vi "调频信号与解调.vi"() -> ()   [LabVIEW 2018]
panel:
  in  "噪声幅度":dbl(slide) min=0.0 max=5.0 scale=0.0..5.0
  out "调制后时域波形":dynamicdata(graph)
  out "发送数据":i32[](array[numeric])
  out "解码正确":bool
  in  "停止":bool
  out "接收数据":dbl[](array[numeric])
  out "滤波后波形":dynamicdata(graph)
  out "相干后波形":dynamicdata(graph)
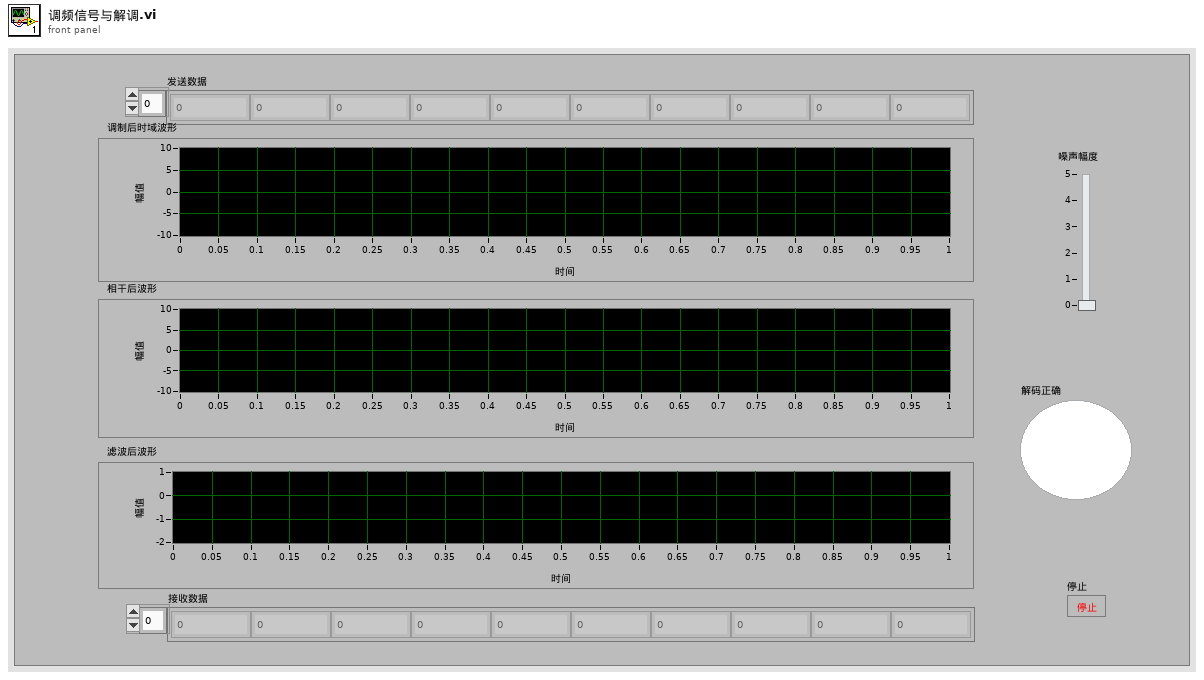
[diagram p1: front panel]
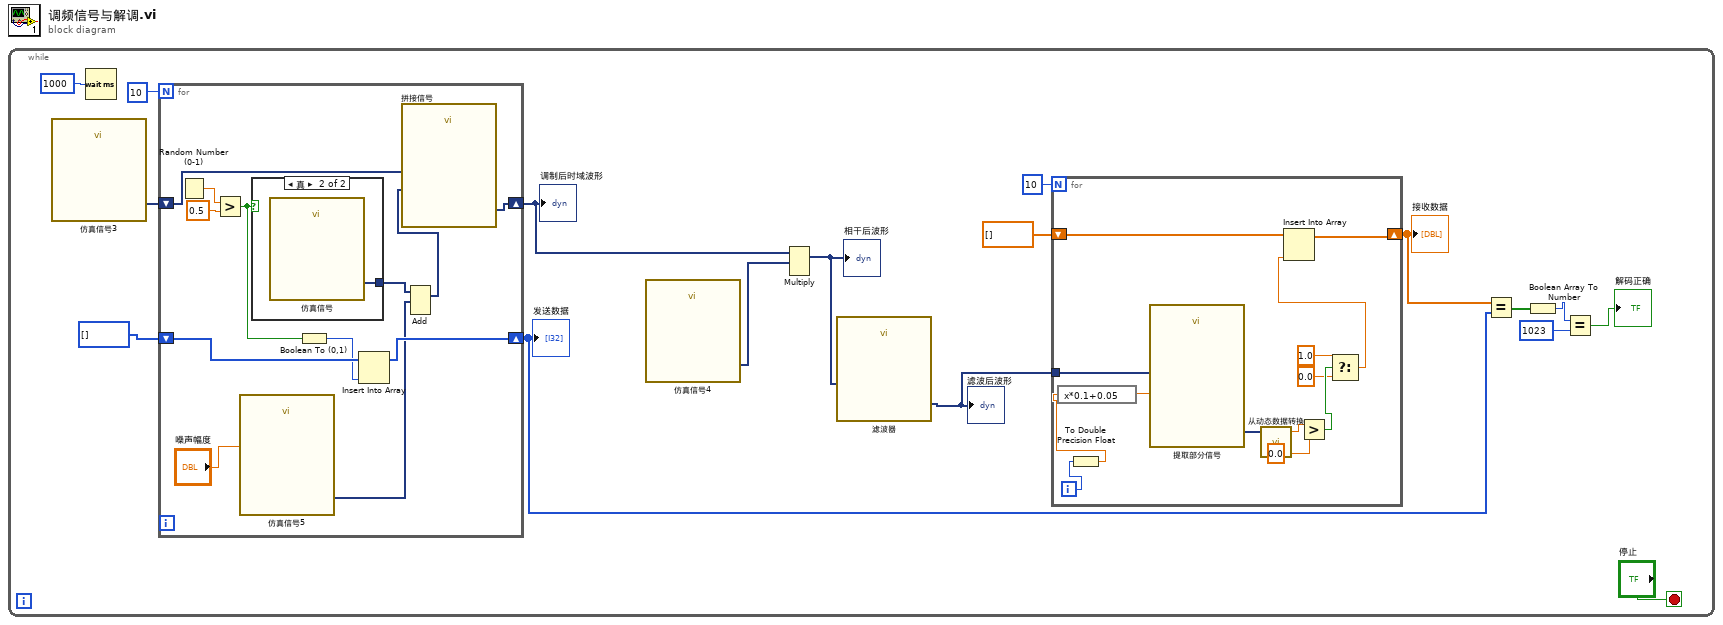
[diagram p0: block diagram]
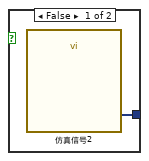
[diagram p2: hidden frame]
diagram:
  n1 = while {
    stop <- "停止" stop-if-true
    n2 = call "仿真信号3"() -> ("正弦"=w16:dynamicdata)  [unwired: 14 in, 1 out]
    n3 = Wait (ms)(milliseconds to wait=u32 1000 ("等待时间（毫秒）")) -> ()  [unwired: 1 out]
    n4 = for {
      N: 10 -> [_]
      shift-right: [w40] -> w11
      shift-left: w16 -> [w39]
      shift-right: [w35] -> w5
      shift-left: i32[] [] -> [w37]
      n5 = Random Number (0-1)() -> (number: 0 to 1=w41:dbl)
      n6 = Greater?(x=w41, y=0.5) -> (0:w38:bool)
      n7 = call "仿真信号5"("噪声幅值"="噪声幅度") -> ("正弦与均匀噪声"=w33:dynamicdata)  [unwired: 13 in, 1 out]
      n8 = case shown="真" w38 {
        tunnel: [w43 w44] -> w32
        frame False {
          n9 = call "仿真信号2"() -> ("正弦"=w43:dynamicdata)  [unwired: 14 in, 1 out]
        }
        frame True {
          n10 = call "仿真信号"() -> ("正弦"=w44:dynamicdata)  [unwired: 14 in, 1 out]
        }
      }
      n11 = Boolean To (0,1)(Boolean=w38) -> (0, 1=w36:i16)
      n12 = Insert Into Array(array=w37, new element=w36) -> (w35:i32[])  [unwired: 1 in]
      n13 = Add(1:w33, 2:w32) -> (0:w31:dynamicdata)  [unwired: 1 in, 1 out]
      n14 = call "拼接信号"("Input Signal B"=w31, "Input Signal A"=w39) -> ("Appended Signals"=w40:dynamicdata)  [unwired: 8 in, 1 out]
    }
    "调制后时域波形" <- w11
    "发送数据" <- w5
    n15 = call "仿真信号4"() -> ("正弦"=w12:dynamicdata)  [unwired: 14 in, 1 out]
    n16 = Multiply(1:w12, 2:w11) -> (0:w10:dynamicdata)  [unwired: 1 in, 1 out]
    "相干后波形" <- w10
    n17 = call "滤波器"("Signal"=w10) -> ("Filtered Signal"=w8:dynamicdata)  [unwired: 9 in, 1 out]
    "滤波后波形" <- w8
    n18 = for {
      N: 10 -> [_]
      tunnel: w8 -> [w30]
      shift-right: [w24] -> w6
      shift-left: dbl[] [] -> [w25]
      i -> [w28]
      n19 = To Double Precision Float(number=w28) -> (double precision float=w27:dbl)
      n20 = expression code="x*0.1+0.05"(w27) -> (w29:dbl)
      n21 = call "提取部分信号"("Begin Offset"=w29, "Signals"=w30) -> ("Section"=w26:dynamicdata)  [unwired: 8 in, 1 out]
      n22 = call "从动态数据转换"("Dynamic Data Type"=w26) -> ("Scalar"=w23:dbl)  [unwired: 3 in]
      n23 = Greater?(x=w23, y=0.0) -> (0:w21:bool)
      n24 = Select(t=1.0, s=w21, f=0.0) -> (s? t:f=w18:dbl)
      n25 = Insert Into Array(array=w25, new element=w18) -> (w24:dbl[])  [unwired: 1 in]
    }
    "接收数据" <- w6
    n26 = Equal?(x=w6, y=w5) -> (x = y?=w4:bool[])
    n27 = Boolean Array To Number(Boolean array=w4) -> (number=w3:u32)
    n28 = Equal?(x=w3, y=u32 1023) -> (x = y?=→"解码正确":bool)
  }
